vi "Find Endpoint Configuration Section.vi"(8 "error in (no error)":errorcluster, 11 "SLSC Switch Custom Device Ref in":T1 format="%.0x") -> (0 "error out":errorcluster, 2 "Endpoint Config Section Ref":T1 format="%.0x", 3 "SLSC Switch Custom Device Ref out":T1 format="%.0x")   [LabVIEW 2017, in "SLSC Switch Scripting.lvlib"]
uses:
  SLSC Switch Scripting.lvlib
  <vilib>/NI Veristand/Custom Device API/Custom Device Item Ref.ctl
  NationalInstruments.VeriStand.SystemDefinitionAPI
  SLSC Scripting Constants.vi
  <vilib>/NI Veristand/Custom Device API/Custom Device API.lvlib
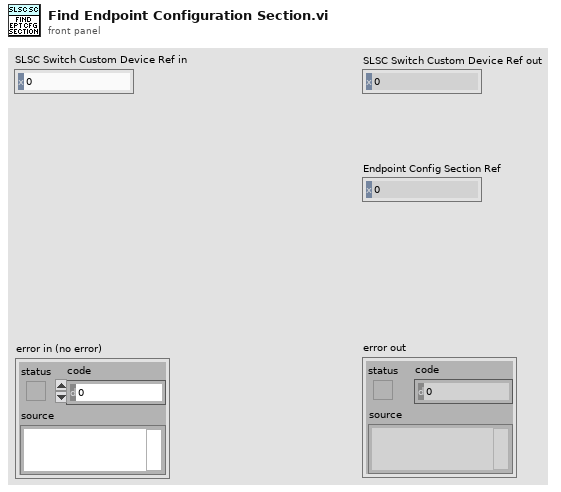
[diagram p1: front panel]
types:
  T1 = typedef "Custom Device API.lvlib/Custom Device Item Ref.ctl" = u64
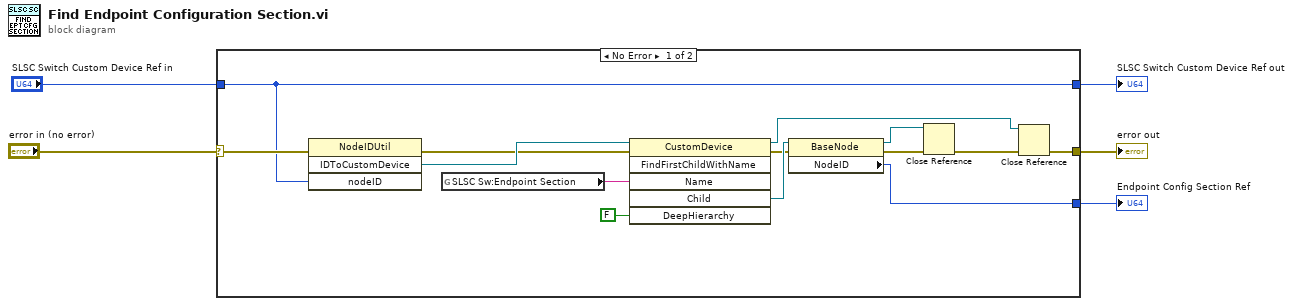
[diagram p0: block diagram]
diagram:
  n1 = case shown="No Error" "error in (no error)" {
    selector: "error in (no error)" -> [w13 w21]
    tunnel: "SLSC Switch Custom Device Ref in" -> [w6 w20]
    tunnel: [w6 w20] -> w4
    tunnel: [w7 w21] -> w3
    tunnel: [w15 _] -> w1
    frame No Error {
      n2 = invoke class="NodeIDUtil" method="IDToCustomDevice"(error in=w13, "nodeID"=w6) -> (error out=w12:errorcluster, "IDToCustomDevice"=w14:refnum<k24>)  [unwired: 2 in, 2 out]
      n3 = global read "SLSC Scripting Constants.vi" "SLSC Sw:Endpoint Section"() -> (w19:string)
      n4 = invoke class="CustomDevice" method="FindFirstChildWithName"(reference=w14, error in=w12, "Name"=w19, "DeepHierarchy"=FALSE) -> (reference out=w8:refnum<k24>, error out=w17:errorcluster, "Child"=w18:refnum<k24>)  [unwired: 2 in, 3 out]
      n5 = property class="BaseNode"(reference=w18, error in=w17) -> (reference out=w10:refnum<k24>, error out=w11:errorcluster, "NodeID"=w15:u64)
      n6 = Close Reference(reference=w10, error in (no error)=w11) -> (error out=w9:errorcluster)
      n7 = Close Reference(reference=w8, error in (no error)=w9) -> (error out=w7:errorcluster)
    }
    frame Error {
    }
  }
  "SLSC Switch Custom Device Ref out" <- w4
  "Endpoint Config Section Ref" <- w1
  "error out" <- w3
